vi "WriteParamsFile.vi"(8 "error in (no error)":errorcluster, 11 ":PmuAnalysis":refnum<class "PmuAnalysis.lvclass">) -> (0 "error out":errorcluster, 3 "PmuAnalysis":refnum<class "PmuAnalysis.lvclass">)   [LabVIEW 2018, in "AnalysisPlugins.lvlib" / "PmuAnalysis.lvclass"]
uses:
  PmuAnalysis.lvclass
  X:/Projects/PMUCal/Modules/Analysis/AnalysisPlugins/AnalysisPluginBaseClass/AnalysisPluginsBase.lvclass
  AnalysisPluginBaseClass/AnalysisPluginsBase.lvclass/AnalysisPluginsBase.ctl
  PmuAnalysis.lvclass/PmuAnalysis.ctl
  FitterBaseClass/Typedefs/clAnalysisConfig.ctl
  AnalysisPluginBaseClass/Accessors/Read AnalysisConfig.vi
  AnalysisPluginBaseClass/Accessors/Read AnalysisTime.vi
  AnalysisPluginBaseClass/Accessors/Read ResultPath.vi
  AnalysisPluginBaseClass/Accessors/Read FileName.vi
  Accessors/Read Function.vi
  Accessors/Read eTestType.vi
  <vilib>/Utility/file.llb/Write Delimited Spreadsheet (string).vi
  FGen/MemberClasses/FunctionBaseClass/FunctionBase.lvclass
  FitterBaseClass/FitterBase.lvclass
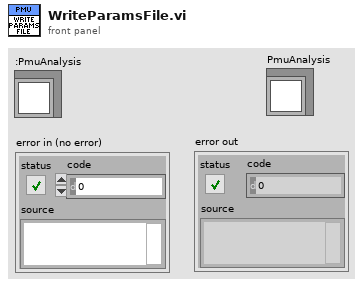
[diagram p1: front panel]
types:
  T1 = typedef "AnalysisPlugins.lvlib/FitterBase.lvclass/clAnalysisConfig.ctl" = cluster{"F0":u32, "SettlingTime":dbl, "AnalysisCycles":dbl, "SampleRate":dbl, "NumChannels":u32, "TsOffset":enum16{"start", "middle", "end"}}
  T2 = enum16{"SteadyState", "Modulation", "Ramp", "Step"}
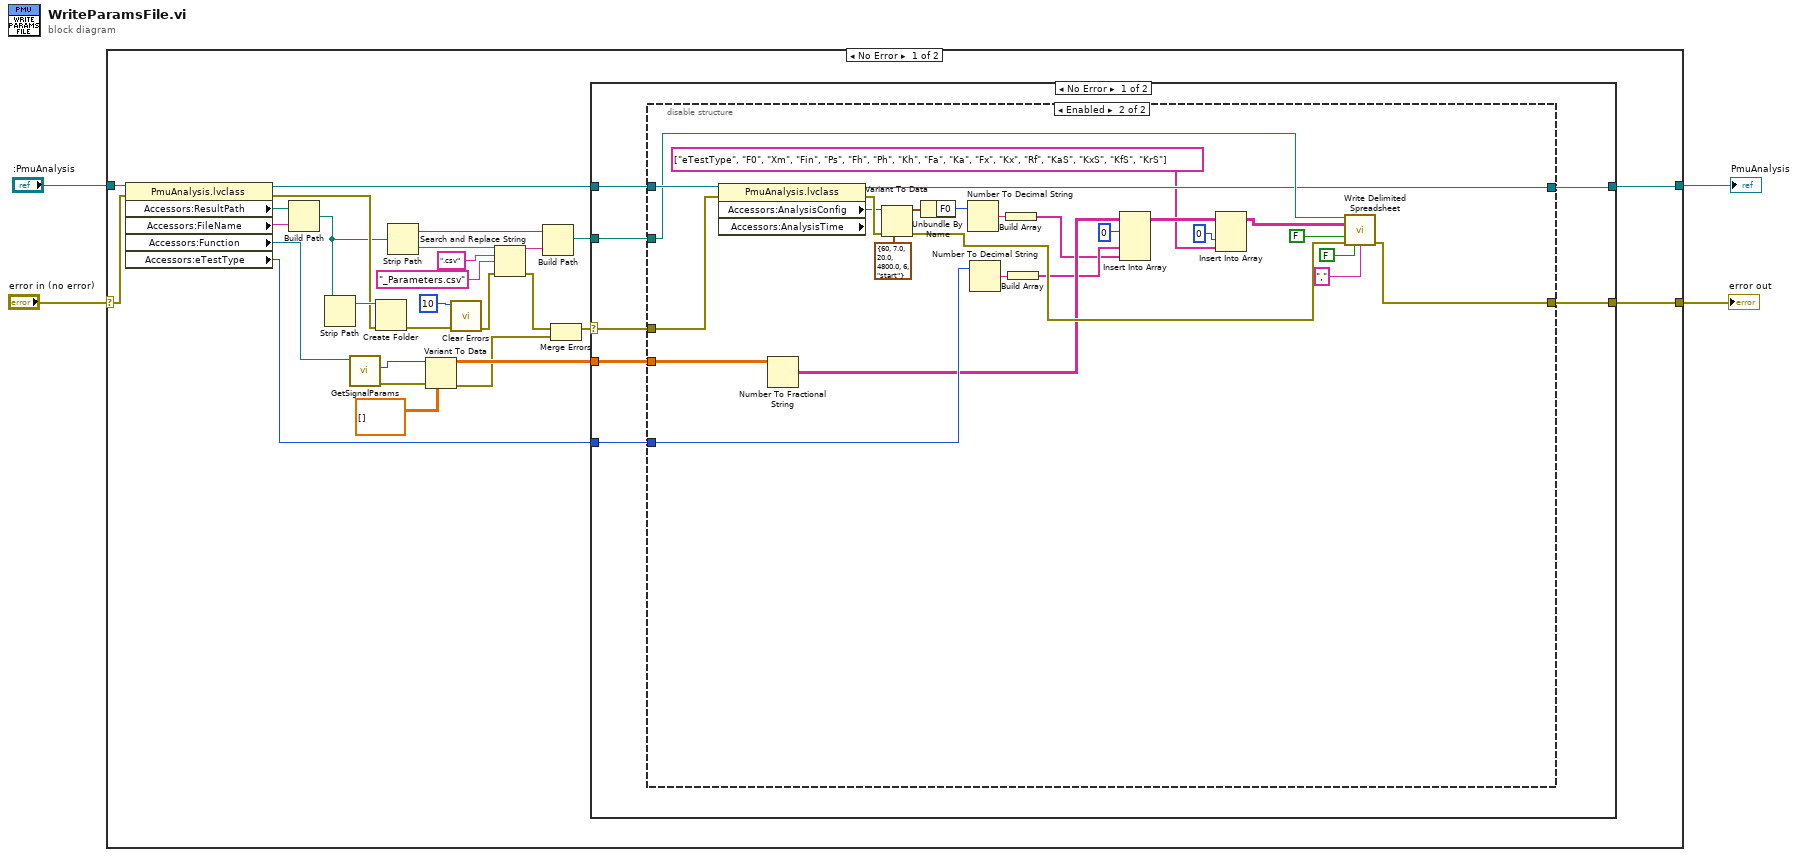
[diagram p0: block diagram]
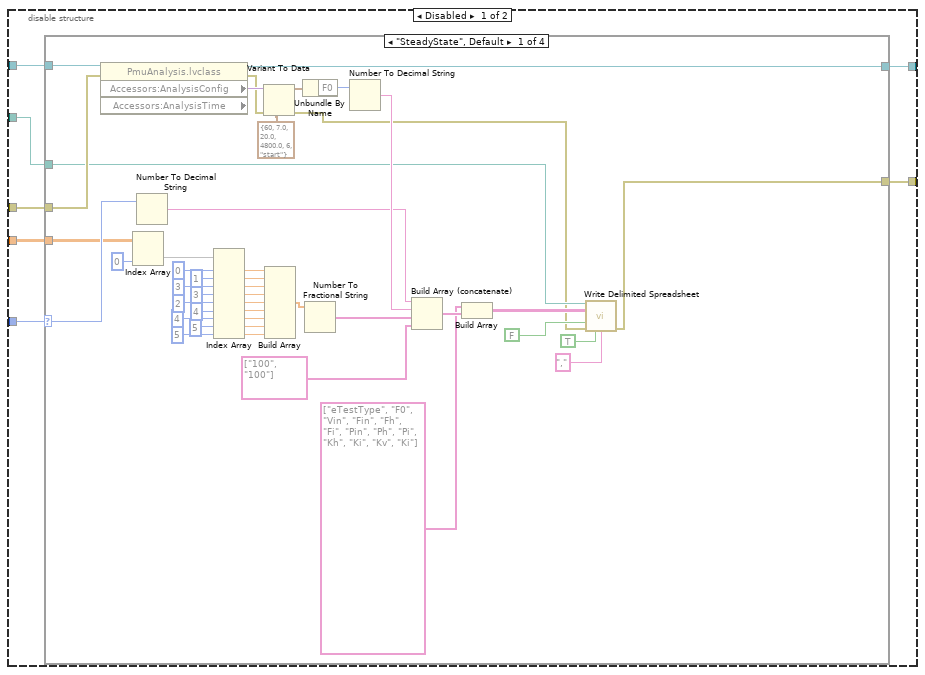
[diagram p2: hidden frame]
diagram:
  n1 = case shown="No Error" "error in (no error)" {
    selector: "error in (no error)" -> [w31 w125]
    tunnel: ":PmuAnalysis" -> [w32 w126]
    tunnel: [w15 w126] -> w1
    tunnel: [w14 w125] -> w2
    frame No Error {
      n2 = property class="PmuAnalysis.lvclass"(reference=w32, error in=w31) -> (reference out=w24:refnum<class "PmuAnalysis.lvclass">, error out=w27:errorcluster, "Accessors:ResultPath"=w30:path, "Accessors:FileName"=w29:string, "Accessors:Function"=w20:refnum<class "FunctionBase.lvclass">, "Accessors:eTestType"=w21:T2)
      n3 = Build Path(base path=w30, name or relative path=w29) -> (appended path=w13:path)
      n4 = Strip Path(path=w13) -> (stripped path=w28:path)  [unwired: 1 out]
      n5 = call-dynamic "GetSignalParams.vi"("FunctionBase in"=w20) -> ("error out"=w23:errorcluster, "Params"=w19:variant)  [unwired: 8 in, 1 out]
      n6 = Create Folder(path (use dialog)=w28, error in=w27) -> (error out=w25:errorcluster)  [unwired: 1 in, 2 out]
      n7 = Strip Path(path=w13) -> (stripped path=w6:path, name=w12:string)
      n8 = Variant To Data(error in=w23, type=dbl[][] [], Variant=w19) -> (data=w18:dbl[][], error out=w16:errorcluster)
      n9 = call <vilib>:"Clear Errors.vi"("error in (no error)"=w25, "specific error code to clear (0: all)"=10) -> ("error out"=w9:errorcluster)  [unwired: 4 in, 1 out]
      n10 = Search and Replace String(input string=w12, search string=".csv" ("substring (\"\")"), replace string="_Parameters.csv" ("substring (\"\")"), error in=w9) -> (result string=w7:string, error out=w8:errorcluster)  [unwired: 4 in, 2 out]
      n11 = Build Path(base path=w6, name or relative path=w7) -> (appended path=w5:path)
      n12 = Merge Errors(w8, w16) -> (w17:errorcluster)
      n13 = case shown="No Error" w17 {
        selector: w17 -> [w36 w123]
        tunnel: w24 -> [w39 w124]
        tunnel: w21 -> [w38 _]
        tunnel: w18 -> [w37 _]
        tunnel: [w34 w124] -> w15
        tunnel: [w33 w123] -> w14
        tunnel: w5 -> [w35 _]
        frame No Error {
          n14 = disable-structure shown="Enabled" {
            disable-tunnel: w39 -> [w46 w116]
            disable-tunnel: w38 -> [w45 w122]
            disable-tunnel: w37 -> [w44 w114]
            disable-tunnel: w36 -> [w43 w115]
            disable-tunnel: w35 -> [w42 w110]
            disable-tunnel: [w41 w109] -> w34
            disable-tunnel: [w40 w107] -> w33
            frame Disabled {
              n15 = case shown="\"SteadyState\", Default" w45 {
                selector: w45 -> [w88 _ _ _]
                tunnel: w43 -> [w89 w91 w93 w95]
                tunnel: w46 -> [w90 w92 w94 w96]
                tunnel: w44 -> [w77 _ _ _]
                tunnel: w42 -> [w53 _ _ _]
                tunnel: [w48 w92 w94 w96] -> w41
                tunnel: [w47 w91 w93 w95] -> w40
                frame "SteadyState", Default {
                  n16 = property class="PmuAnalysis.lvclass" props=["Accessors:AnalysisConfig", "Accessors:AnalysisTime"](reference=w90, error in=w89) -> (reference out=w48:refnum<class "PmuAnalysis.lvclass">, error out=w72:errorcluster, "Accessors:AnalysisConfig"=w73:variant)  [unwired: 1 out]
                  n17 = Index Array(array=w77, index (col)=0 ("disabled index (col)")) -> (element=w75:dbl[])  [unwired: 1 in]
                  n18 = Number To Decimal String(number=w88) -> (decimal integer string=w58:string)  [unwired: 1 in]
                  n19 = Index Array(array=w75, index #1=0 ("index"), index #2=1 ("index"), index #3=3 ("index"), index #4=3 ("index"), index #5=2 ("index"), index #6=4 ("index"), index #7=4 ("index"), index #8=5 ("index"), index #9=5 ("index")) -> (element #1=w87:dbl, element #2=w86:dbl, element #3=w85:dbl, element #4=w84:dbl, element #5=w83:dbl, element #6=w82:dbl, element #7=w79:dbl, element #8=w80:dbl, element #9=w81:dbl)
                  n20 = Variant To Data(error in=w72, type=T1 {"F0"=60, "SettlingTime"=7.0, "AnalysisCycles"=20.0, "SampleRate"=4800.0, "NumChannels"=6, "TsOffset"=enum."start"} ("clAnalysisConfig"), Variant=w73) -> (data=w70:T1, error out=w51:errorcluster)
                  n21 = Build Array(w87, w86, w85, w84, w83, w82, w79, w80, w81) -> (w78:dbl[])
                  n22 = Unbundle By Name(w70) -> ("F0"=w69:u32)
                  n23 = Number To Fractional String(number=w78) -> (F-format string=w74:string[])  [unwired: 3 in]
                  n24 = Number To Decimal String(number=w69) -> (decimal integer string=w68:string)  [unwired: 1 in]
                  n25 = Build Array (concatenate)(w58, w68, w74, string[] ["100", "100"]) -> (w56:string[])
                  n26 = Build Array(string[] ["eTestType", "F0", "Vin", "Fin", "Fh", "Fi", "Pin", "Ph", "Pi", "Kh", "Ki", "Kv", "Ki"], w56) -> (w54:string[][])
                  n27 = call-poly <vilib>:"Write Delimited Spreadsheet.vi"("file path (dialog if empty)"=w53, "2D data"=w54, "append to file? (new file:F)"=FALSE, "error in (no error)"=w51, "transpose? (no:F)"=TRUE, "delimiter (\\t)"="," ("delimiter (\\t)")) -> ("error out"=w47:errorcluster)  [unwired: 8 in, 1 out]
                }
                frame "Modulation" {
                }
                frame "Ramp" {
                }
                frame "Step" {
                }
              }
            }
            frame Enabled {
              n28 = property class="PmuAnalysis.lvclass" props=["Accessors:AnalysisConfig", "Accessors:AnalysisTime"](reference=w116, error in=w115) -> (reference out=w109:refnum<class "PmuAnalysis.lvclass">, error out=w119:errorcluster, "Accessors:AnalysisConfig"=w118:variant)  [unwired: 1 out]
              n29 = Number To Fractional String(number=w114) -> (F-format string=w106:string[][])  [unwired: 3 in]
              n30 = Variant To Data(error in=w119, type=T1 {"F0"=60, "SettlingTime"=7.0, "AnalysisCycles"=20.0, "SampleRate"=4800.0, "NumChannels"=6, "TsOffset"=enum."start"} ("clAnalysisConfig"), Variant=w118) -> (data=w120:T1, error out=w108:errorcluster)
              n31 = Unbundle By Name(w120) -> ("F0"=w121:u32)
              n32 = Number To Decimal String(number=w121) -> (decimal integer string=w104:string)  [unwired: 1 in]
              n33 = Number To Decimal String(number=w122) -> (decimal integer string=w103:string)  [unwired: 1 in]
              n34 = Build Array(w104) -> (w101:string[])
              n35 = Build Array(w103) -> (w102:string[])
              n36 = Insert Into Array(array=w106, index (row)=0 ("disabled index (col)"), new element #1=w102, new element #2=w101) -> (w100:string[][])  [unwired: 1 in]
              n37 = Insert Into Array(array=w100, index (col)=0 ("disabled index (col)"), new element=string[] ["eTestType", "F0", "Xm", "Fin", "Ps", "Fh", "Ph", "Kh", "Fa", "Ka", "Fx", "Kx", "Rf", "KaS", "KxS", "KfS", "KrS"]) -> (w99:string[][])  [unwired: 1 in]
              n38 = call-poly <vilib>:"Write Delimited Spreadsheet.vi"("file path (dialog if empty)"=w110, "2D data"=w99, "append to file? (new file:F)"=FALSE, "error in (no error)"=w108, "transpose? (no:F)"=FALSE, "delimiter (\\t)"="," ("delimiter (\\t)")) -> ("error out"=w107:errorcluster)  [unwired: 8 in, 1 out]
            }
          }
        }
        frame Error {
        }
      }
    }
    frame Error {
    }
  }
  "PmuAnalysis" <- w1
  "error out" <- w2
